vi "To XML - Id defined - XML contains id.vi"() -> ()   [LabVIEW 2013, in "JUnit XML Tests.lvlib" / "Test Suite.lvlib"]
uses:
  Test Suite.lvlib
  JUnit XML/Test Suite/Test Suite.lvclass/Test Suite.ctl
  JUnit XML/Test Suite/Test Suite.lvclass
  JUnit XML/Test Suite/Write Timestamp.vi
  <vilib>/xml/Close Reference(Node).vi
  <vilib>/addons/_JKI Toolkits/Caraya/classes/Assert/Assert Equal Value_Variant.vi
  JUnit XML/JUnit XML.lvlib
  <vilib>/addons/_JKI Toolkits/Caraya/classes/Test/Test.lvclass
  <vilib>/addons/_JKI Toolkits/Caraya/classes/Assert/Assert.lvclass
  <resource>/objmgr/DOMUserDefRef.rc
  <vilib>/xml/NI_XML.lvlib
panel:
  out "error out":errorcluster
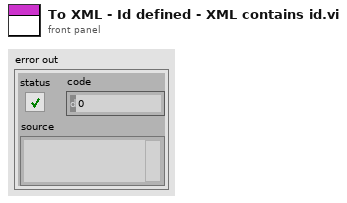
[diagram p1: front panel]
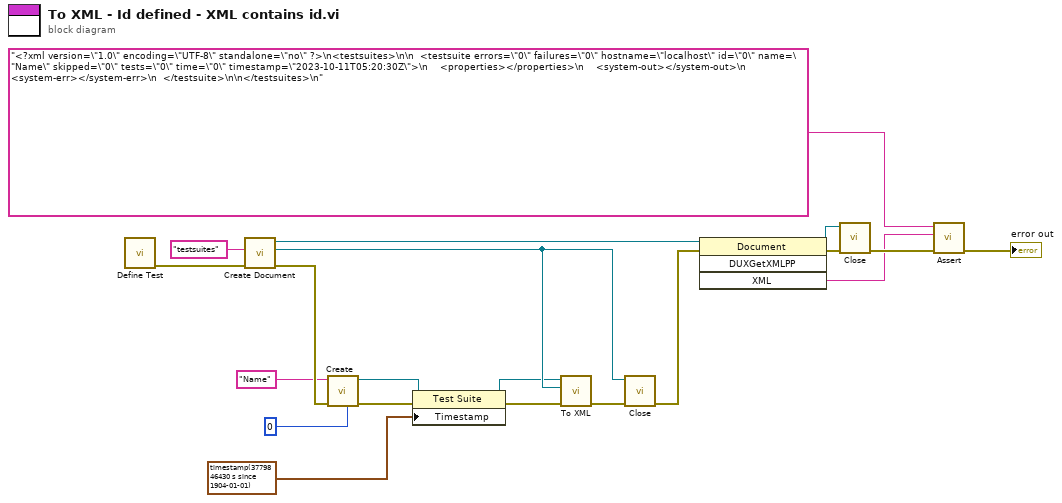
[diagram p0: block diagram]
diagram:
  n1 = call <vilib>:"Define Test.vi"() -> ("error out"=w20:errorcluster)  [unwired: 10 in, 1 out]
  n2 = call "Create Document.vi"("error in (no error)"=w20, "Root Element Name"="testsuites") -> ("error out"=w17:errorcluster, "Root Element"=w13:refnum<k20>, "Document"=w16:refnum<k20>)  [unwired: 7 in]
  n3 = call "Create.vi"("Id (-1 = undefined)"=0, "error in (no error)"=w17, "Name"="Name" ("Package")) -> ("error out"=w19:errorcluster, "Test Suite"=w5:refnum<class "Test Suite.lvclass">)  [unwired: 7 in]
  n4 = property class="Test Suite"(reference=w5, error in=w19, "Timestamp"=timestamp(3779846430.123 s since 1904-01-01)) -> (reference out=w4:refnum<class "Test Suite.lvclass">, error out=w6:errorcluster)
  n5 = call-dynamic "To XML.vi"("error in (no error)"=w6, "Parent"=w13, "Test Suite in"=w4) -> ("error out"=w15:errorcluster)  [unwired: 8 in]
  n6 = call-poly <vilib>:"Close.vi"("error in (no error)"=w15, "node"=w13) -> ("error out"=w14:errorcluster)  [unwired: 7 in]
  n7 = invoke class="Document" method="DUXGetXMLPP"(reference=w16, error in=w14) -> (reference out=w11:refnum<k20>, error out=w12:errorcluster, "XML"=w9:string)  [unwired: 2 in, 1 out]
  n8 = call-poly <vilib>:"Close.vi"("error in (no error)"=w12, "node"=w11) -> ("error out"=w10:errorcluster)  [unwired: 7 in]
  n9 = call-poly <vilib>:"Assert.vi"("error in (no error)"=w10, "Actual"=w9, "Expected"="<?xml version=\"1.0\" encoding=\"UTF-8\" standalone=\"no\" ?>\n<testsuites>\n\n  <testsuite errors=\"0\" failures=\"0\" hostname=\"localhost\" id=\"0\" name=\"Name\" skipped=\"0\" tests=\"0\" time=\"0\" timestamp=\"2023-10-11T05:20:30Z\">\n    <properties></properties>\n    <system-out></system-out>\n    <system-err></system-err>\n  </testsuite>\n\n</testsuites>\n") -> ("error out"=→"error out":errorcluster)  [unwired: 7 in, 1 out]
